vi "Manual Assembly.vi"() -> ()   [LabVIEW 2018]
uses:
  Classes/Assembly/Assembly Run.lvclass
  Classes/Controller/Controller.lvclass
  Classes/Workspace/Fixture Enum.ctl
  Classes/Workspace/Fixture.lvclass
  Classes/Routine/Routine Enum.ctl
  Classes/Routine/Routine.lvclass
panel:
  in  "Clear All":bool
  in  "Assemble":bool
  in  "Dispense offset":bool
  in  "Pick and Place":bool
  in  "Dispense glue":bool
  in  "Gantry":T1
  in  "Go":bool
  in  "Routine":T2=enum."Dispense on Plate"
  in  "Update":bool
  in  "Stage":i32(listbox)=-1
  in  "Stop":bool
  in  "Remove":bool
  in  "Add":bool
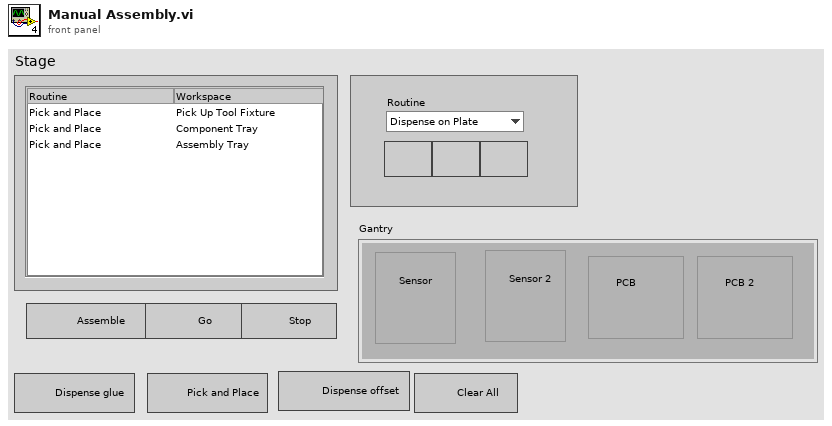
[diagram p1: front panel]
types:
  T1 = cluster{"Sensor":bool, "Sensor 2":bool, "PCB":bool, "PCB 2":bool}
  T2 = typedef "Routine.lvclass/Routine Enum.ctl" = enum16{"Primary Pick Up", "Pick Up All", "Put Down Secondary", "Put Down All", "Release Syringe", "Secondary Pick Up", "Secure Syringe", "Dispense on Plate", "Dispense on Kapton", "Dispense on Sensor"}
  T3 = typedef "Fixture.lvclass/Fixture Enum.ctl" = enum16{"Assembly Tray", "Syringe Space", "Component", "Pick Up Tool", "Current Position"}
  T4 = cluster{"[0]":bool, "[1]":bool, "[2]":bool, "[3]":bool}
  T5 = typedef "Controller.lvclass/Controllers.ctl" = cluster{"I-O.lvclass":refnum<class "I-O.lvclass">, "Gantry":refnum<k24>, "Dispenser":refnum<visa-resource-name>}
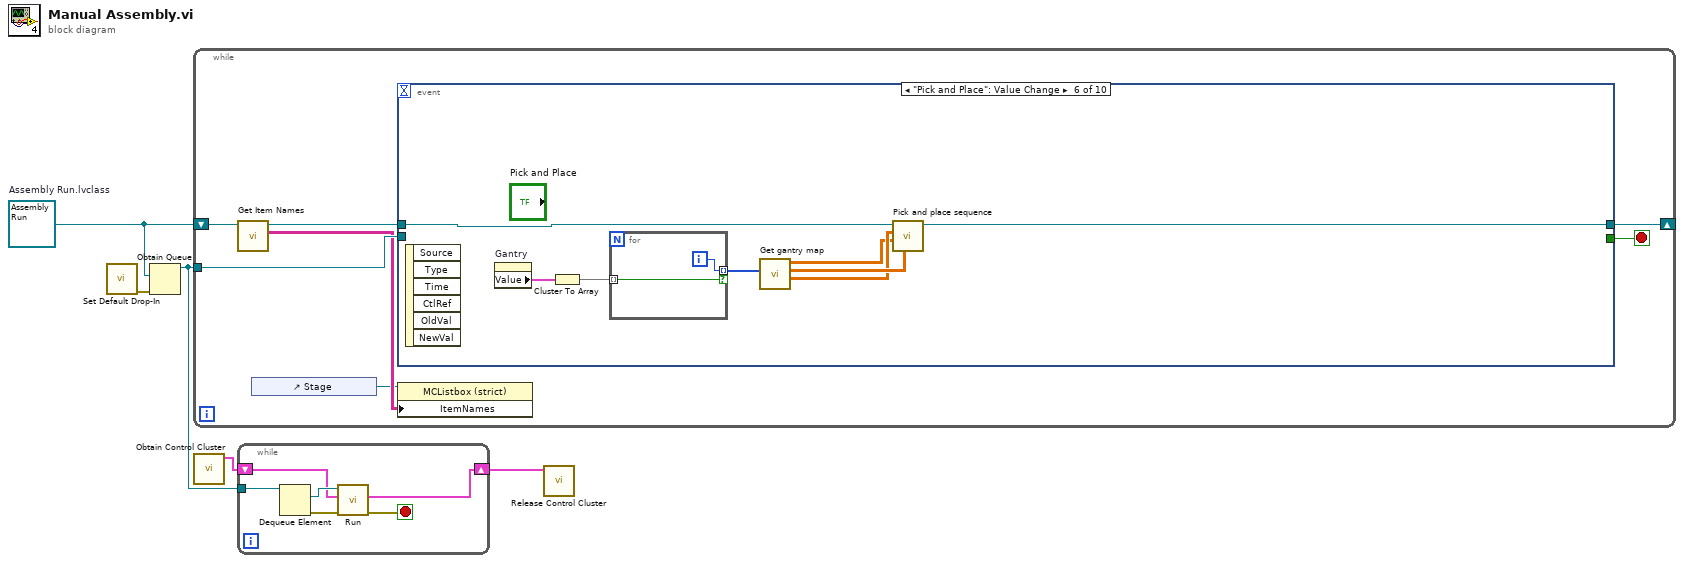
[diagram p0: block diagram]
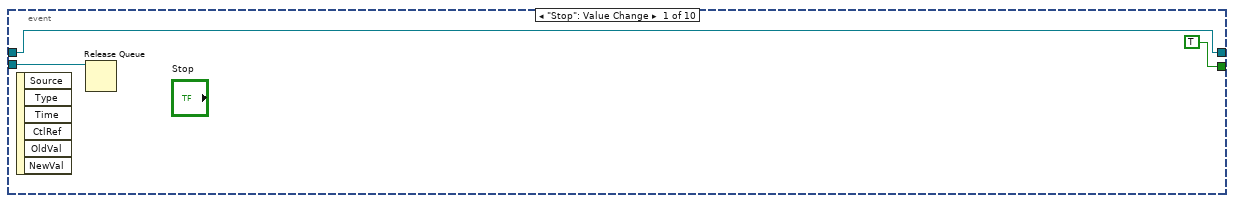
[diagram p2: hidden frame]
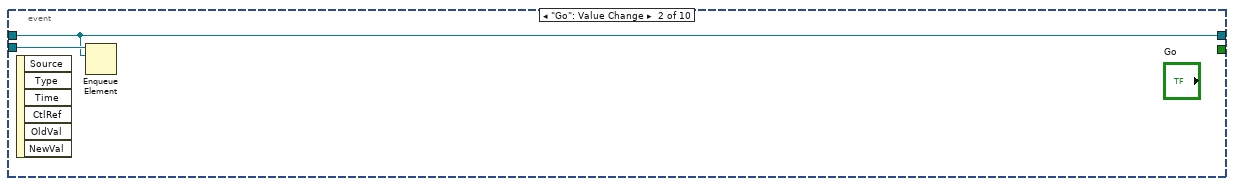
[diagram p3: hidden frame]
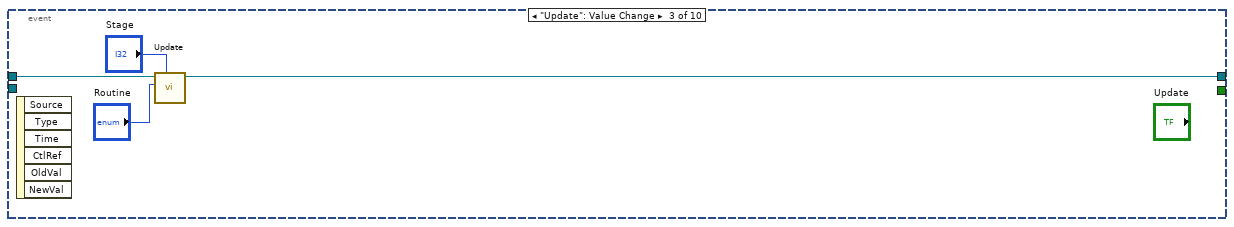
[diagram p4: hidden frame]
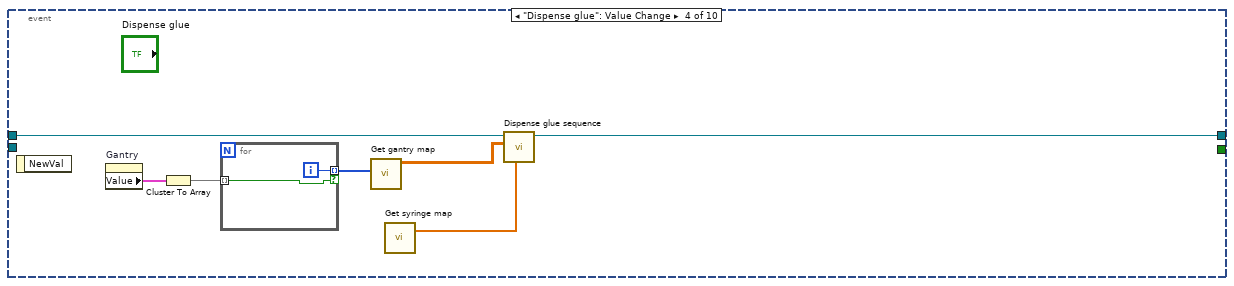
[diagram p5: hidden frame]
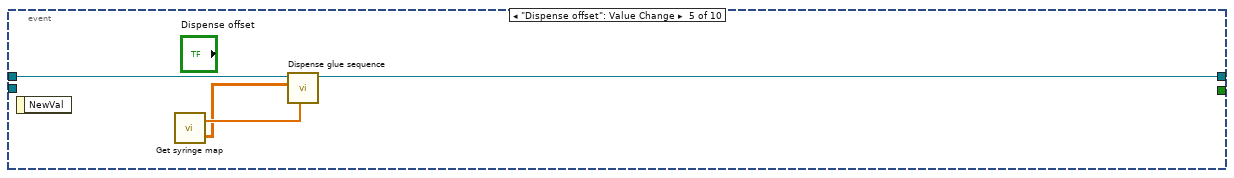
[diagram p6: hidden frame]
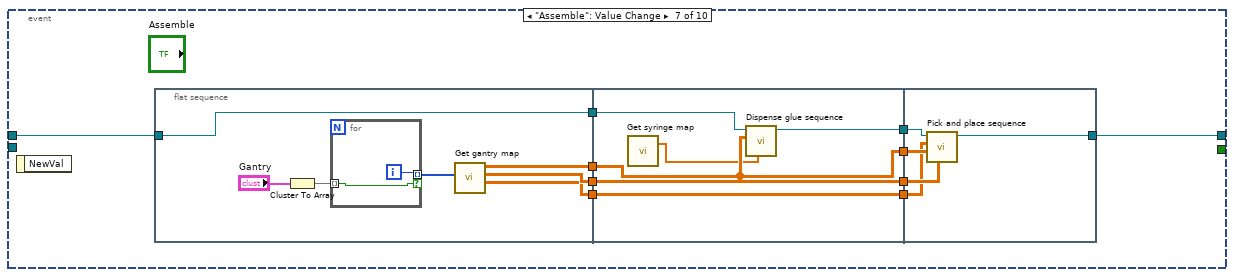
[diagram p7: hidden frame]
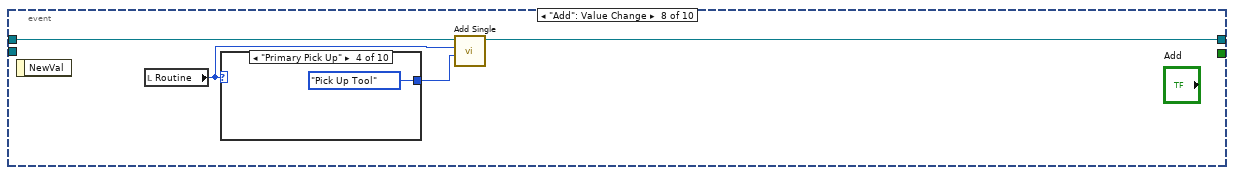
[diagram p8: hidden frame]
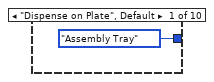
[diagram p9: hidden frame]
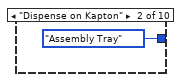
[diagram p10: hidden frame]
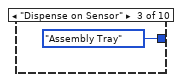
[diagram p11: hidden frame]
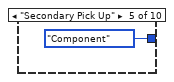
[diagram p12: hidden frame]
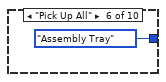
[diagram p13: hidden frame]
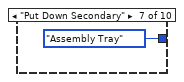
[diagram p14: hidden frame]
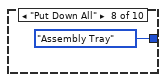
[diagram p15: hidden frame]
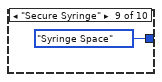
[diagram p16: hidden frame]
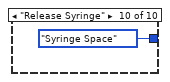
[diagram p17: hidden frame]
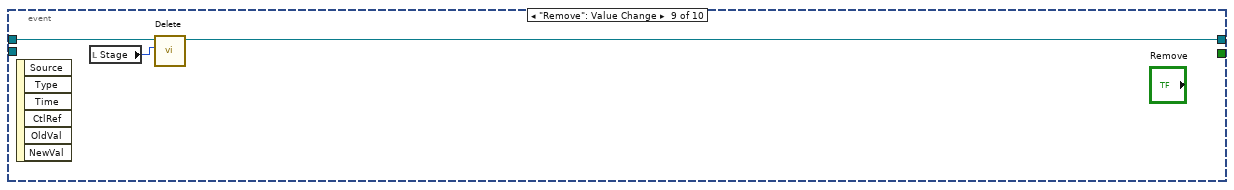
[diagram p18: hidden frame]
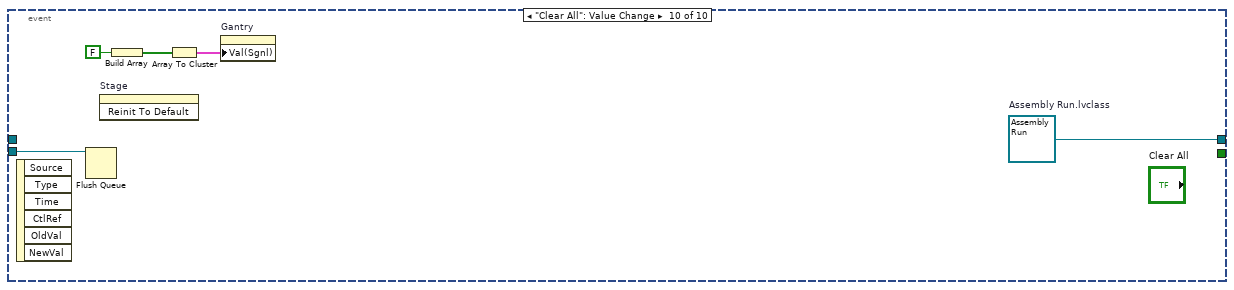
[diagram p19: hidden frame]
diagram:
  w2 = refnum<class "Assembly Run.lvclass"> refnum  # Assembly Run.lvclass
  n1 = call "Set Default Drop-In.vi"() -> ("error out"=w3:errorcluster)  [unwired: 11 in]
  n2 = Obtain Queue(element data type=w2, error in (no error)=w3) -> (queue out=w5:refnum<queue>)  [unwired: 3 in, 2 out]
  n3 = while {
    shift-right: [w6] -> _
    shift-left: w2 -> [w8]
    tunnel: w5 -> [w11]
    stop <- w12 stop-if-true
    n4 = call "Get Item Names.vi"("Assembly Run in"=w8) -> ("Item names"=w10:string[][], "Assembly Run out"=w7:refnum<class "Assembly Run.lvclass">)  [unwired: 8 in, 1 out]
    n5 = control-ref of="Stage"() -> (w9:refnum<vi>)
    n6 = event shown="[5] \"Pick and Place\": Value Change" {
      selector: _ -> [_ _ _ _ _ _ _ _ _ _]
      dyn-events: _ -> [_ _ _ _ _ _ _ _ _ _]
      timeout: _ -> [_ _ _ _ _ _ _ _ _ _]
      tunnel: [TRUE _ _ _ _ _ _ _ _ _] -> w12
      tunnel: w7 -> [w14 w16 w21 w27 w34 w41 w54 w77 w91 _]
      tunnel: [w14 w16 w20 w25 w33 w40 w53 w76 w90 w96] -> w6
      tunnel: w11 -> [w13 w17 _ _ _ _ _ _ _ w95]
      event "Stop": Value Change {
        n7 = event-data() -> ()  [unwired: 1 in, 6 out]
        n8 = Release Queue(queue=w13) -> ()  [unwired: 2 in, 3 out]
      }
      event "Go": Value Change {
        n9 = event-data() -> ()  [unwired: 1 in, 6 out]
        n10 = Enqueue Element(queue=w17, element=w16) -> ()  [unwired: 2 in, 3 out]
      }
      event "Update": Value Change {
        n11 = event-data() -> ()  [unwired: 1 in, 6 out]
        n12 = call "Update.vi"("Row"="Stage", "Routine"="Routine", "Assembly Run in"=w21) -> ("Assembly Run out"=w20:refnum<class "Assembly Run.lvclass">)  [unwired: 7 in, 1 out]
      }
      event "Dispense glue": Value Change {
        n13 = event-data() -> ()  [unwired: 1 in, 1 out]
        n14 = property on="Gantry" class="Clust (strict)"() -> ("Value"=w23:T1)  [unwired: 2 in, 2 out]
        n15 = Cluster To Array(cluster=w23) -> (array=w24:bool[])
        n16 = for {
          tunnel: w24 -> [w29] mode=indexing
          tunnel: [w30] -> w28 mode=indexing if=w29
          i -> [w30]
        }
        n17 = call "Get gantry map.vi"("Selection Array"=w28) -> ("Assembly Tray map"=w26:dbl[][])  [unwired: 8 in, 2 out]
        n18 = call "Get syringe map.vi"() -> ("Syringe map"=w22:dbl[])  [unwired: 2 in, 1 out]
        n19 = call "Dispense glue sequence.vi"("Syringe map"=w22, "Assembly Tray map"=w26, "Assembly Run in"=w27) -> ("Assembly Run out"=w25:refnum<class "Assembly Run.lvclass">)  [unwired: 7 in, 1 out]
      }
      event "Dispense offset": Value Change {
        n20 = event-data() -> ()  [unwired: 1 in, 1 out]
        n21 = call "Get syringe map.vi"() -> ("Offset map (2D 1 row)"=w31:dbl[][], "Syringe map"=w32:dbl[])  [unwired: 2 in]
        n22 = call "Dispense glue sequence.vi"("Syringe map"=w32, "Assembly Tray map"=w31, "Assembly Run in"=w34) -> ("Assembly Run out"=w33:refnum<class "Assembly Run.lvclass">)  [unwired: 7 in, 1 out]
      }
      event "Pick and Place": Value Change {
        n23 = event-data() -> ()  [unwired: 1 in, 6 out]
        n24 = property on="Gantry" class="Clust (strict)"() -> ("Value"=w37:T1)  [unwired: 2 in, 2 out]
        n25 = Cluster To Array(cluster=w37) -> (array=w38:bool[])
        n26 = for {
          tunnel: w38 -> [w43] mode=indexing
          tunnel: [w44] -> w42 mode=indexing if=w43
          i -> [w44]
        }
        n27 = call "Get gantry map.vi"("Selection Array"=w42) -> ("PUT map"=w36:dbl[][], "Component Tray map"=w39:dbl[][], "Assembly Tray map"=w35:dbl[][])  [unwired: 8 in]
        n28 = call "Pick and place sequence.vi"("Component Tray map"=w39, "Assembly Tray map"=w35, "PUT map"=w36, "Assembly Run in"=w41) -> ("Assembly Run out"=w40:refnum<class "Assembly Run.lvclass">)  [unwired: 6 in, 1 out]
      }
      event "Assemble": Value Change {
        n29 = event-data() -> ()  [unwired: 1 in, 1 out]
        n30 = flat-sequence {
          tunnel: w54 -> [w61]
          tunnel: [w61] -> w51
          tunnel: [w57] -> w50
          tunnel: [w56] -> w47
          tunnel: [w55] -> w45
          tunnel: [w68] -> w52
          tunnel: w51 -> [w69]
          tunnel: w50 -> [w67]
          tunnel: [w67] -> w49
          tunnel: [w66] -> w48
          tunnel: w47 -> [w66]
          tunnel: [w65] -> w46
          tunnel: w45 -> [w65]
          tunnel: [w73] -> w53
          tunnel: w52 -> [w74]
          tunnel: w49 -> [w72]
          tunnel: w48 -> [w71]
          tunnel: w46 -> [w70]
          frame #0 {
            n31 = Cluster To Array(cluster="Gantry") -> (array=w60:bool[])
            n32 = for {
              tunnel: w60 -> [w62] mode=indexing
              tunnel: [w63] -> w58 mode=indexing if=w62
              i -> [w63]
            }
            n33 = call "Get gantry map.vi"("Selection Array"=w58) -> ("PUT map"=w55:dbl[][], "Component Tray map"=w56:dbl[][], "Assembly Tray map"=w57:dbl[][])  [unwired: 8 in]
          }
          frame #1 {
            n34 = call "Get syringe map.vi"() -> ("Syringe map"=w64:dbl[])  [unwired: 2 in, 1 out]
            n35 = call "Dispense glue sequence.vi"("Syringe map"=w64, "Assembly Tray map"=w67, "Assembly Run in"=w69) -> ("Assembly Run out"=w68:refnum<class "Assembly Run.lvclass">)  [unwired: 7 in, 1 out]
          }
          frame #2 {
            n36 = call "Pick and place sequence.vi"("Component Tray map"=w71, "Assembly Tray map"=w72, "PUT map"=w70, "Assembly Run in"=w74) -> ("Assembly Run out"=w73:refnum<class "Assembly Run.lvclass">)  [unwired: 6 in, 1 out]
          }
        }
      }
      event "Add": Value Change {
        n37 = event-data() -> ()  [unwired: 1 in, 1 out]
        n38 = local read "Routine"() -> (w75:T2)
        n39 = case shown="\"Primary Pick Up\"" w75 {
          tunnel: [Fixture_Enum."Assembly Tray" ("Fixture") Fixture_Enum."Assembly Tray" ("Fixture") Fixture_Enum."Assembly Tray" ("Fixture") Fixture_Enum."Pick Up Tool" ("Fixture") Fixture_Enum."Component" ("Fixture") Fixture_Enum."Assembly Tray" ("Fixture") Fixture_Enum."Assembly Tray" ("Fixture") Fixture_Enum."Assembly Tray" ("Fixture") Fixture_Enum."Syringe Space" ("Fixture") Fixture_Enum."Syringe Space" ("Fixture")] -> w78
          frame "Dispense on Plate", Default {
          }
          frame "Dispense on Kapton" {
          }
          frame "Dispense on Sensor" {
          }
          frame "Primary Pick Up" {
          }
          frame "Secondary Pick Up" {
          }
          frame "Pick Up All" {
          }
          frame "Put Down Secondary" {
          }
          frame "Put Down All" {
          }
          frame "Secure Syringe" {
          }
          frame "Release Syringe" {
          }
        }
        n40 = call-dynamic "Add Single.vi"("Fixture"=w78, "Routine"=w75, "UI in"=w77) -> ("UI out"=w76:refnum<class "Assembly Run.lvclass">)  [unwired: 6 in, 1 out]
      }
      event "Remove": Value Change {
        n41 = event-data() -> ()  [unwired: 1 in, 6 out]
        n42 = local read "Stage"() -> (w89:i32)
        n43 = call "Delete.vi"("Index"=w89, "Assembly In"=w91) -> ("Assembly Out"=w90:refnum<class "Assembly Run.lvclass">)  [unwired: 8 in, 1 out]
      }
      event "Clear All": Value Change {
        w96 = refnum<class "Assembly Run.lvclass"> refnum  # Assembly Run.lvclass
        n44 = event-data() -> ()  [unwired: 1 in, 6 out]
        n45 = Flush Queue(queue=w95) -> ()  [unwired: 1 in, 3 out]
        n46 = invoke on="Stage" class="MCListbox (strict)" method="Reinit To Default"() -> ()  [unwired: 3 in, 3 out]
        n47 = Build Array(FALSE) -> (w93:bool[])
        n48 = Array To Cluster(array=w93) -> (cluster=w94:T4)
        n49 = property on="Gantry" class="Clust (strict)"("Val(Sgnl)"=w94) -> ()  [unwired: 2 in, 2 out]
      }
    }
    n50 = property class="MCListbox (strict)"(reference=w9, "ItemNames"=w10) -> ()  [unwired: 1 in, 2 out]
  }
  n51 = call "Obtain Control Cluster.vi"() -> ("Control Out"=w1:T5)  [unwired: 11 in]
  n52 = while {
    tunnel: w5 -> [w102]
    shift-right: [w97] -> w4
    shift-left: w1 -> [w98]
    stop <- w99 stop-if-true
    n53 = Dequeue Element(queue=w102) -> (element=w101:refnum<class "Assembly Run.lvclass">, error out=w100:errorcluster)  [unwired: 2 in, 2 out]
    n54 = call-dynamic "Run.vi"("error in (no error)"=w100, "Control In"=w98, "Assembly In"=w101) -> ("error out"=w99:errorcluster, "Control Out"=w97:T5)  [unwired: 6 in, 1 out]
  }
  n55 = call "Release Control Cluster.vi"("output cluster"=w4) -> ()  [unwired: 11 in]
